vi "Send Pre-Addressed Subscribe.vi"(8 "error in (no error)":errorcluster, 10 "Subscription Request":refnum<class "SubscriptionRequest.lvclass">, 11 "Subscribe Msg":refnum<class "Subscribe Msg.lvclass">) -> (0 "error out":errorcluster)   [LabVIEW 2020, in "IMediator.lvlib" / "Subscribe Msg.lvclass"]
doc: "发送订阅消息"
uses:
  Subscribe Msg.lvclass
  SubscriptionRequest/SubscriptionRequest.lvclass
  Subscribe Msg.lvclass/Subscribe Msg.ctl
  composed-af-messages/Source/RoundTripMessage/RoundTripMessage.lvclass/RoundTripMessage.ctl
  <vilib>/ActorFramework/Message Enqueuer/Message Enqueuer.lvclass/Message Enqueuer.ctl
  <vilib>/ActorFramework/Message Enqueuer/Enqueue.vi
  composed-af-messages/Source/RoundTripMessage/RoundTripMessage.lvclass
  C:/Program Files/National Instruments/LabVIEW 2020/vi.lib/ActorFramework/Message/Message.lvclass
  <vilib>/ActorFramework/Message Priority Queue/Priority Enqueue.vi
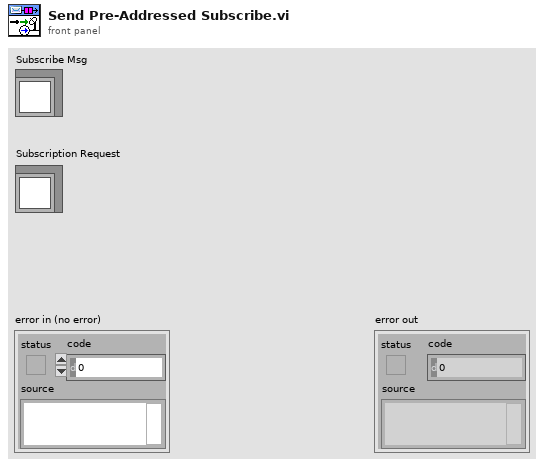
[diagram p1: front panel]
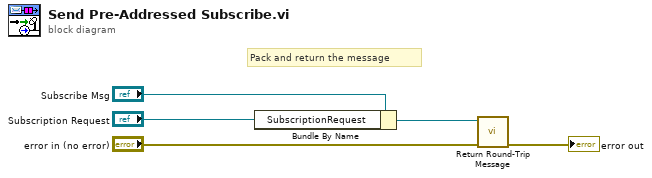
[diagram p0: block diagram]
diagram:
  # "Pack and return the message"
  n1 = Bundle By Name(cluster="Subscribe Msg", "SubscriptionRequest"="Subscription Request") -> (w2:refnum<class "Subscribe Msg.lvclass">)
  n2 = call "Return Round-Trip Message.vi"("error in (no error)"="error in (no error)", "RoundTripMessage In"=w2) -> ("error out"=→"error out":errorcluster)  [unwired: 9 in]
